vi "探头窗口-6.vi"() -> ()   [LabVIEW 2017]
panel:
  in  "更新数据":T1
  in  "停止信号":bool=TRUE
  out "更新数据？":bool=TRUE
  out "引用-切回列表模式？":refnum<vi>
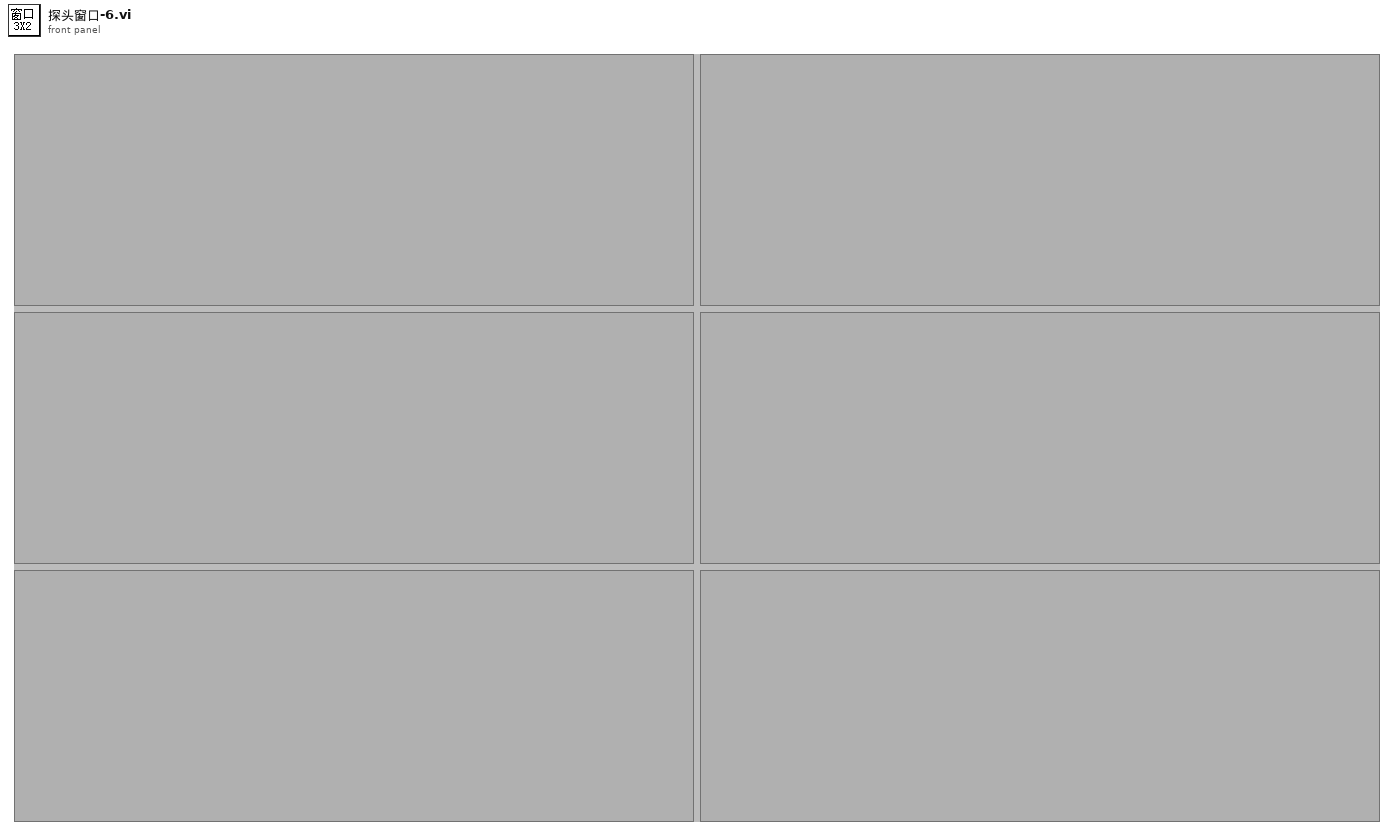
[diagram p1: front panel]
types:
  T1 = cluster{"探头启用状态？":bool[], "测量值":cluster{"X":timestamp, "Y":dbl}[], "限值":cluster{"限值1":dbl, "限值2":dbl, "探头限值":enum16{"一级限值", "二级限值"}}[], "报警状态":enum16{"正常", "一级报警", "二级报警", "累积报警"}[], "探头信息":string[], "累积剂量":cluster{"设备名称":string, "启用累积？":bool, "起始时间":timestamp, "累积剂量":dbl, "累积报警阈值":dbl}[]}
  T2 = cluster{"启用状态？":bool, "测量值":cluster{"X":timestamp, "Y":dbl}, "限值簇":cluster{"限值1":dbl, "限值2":dbl, "探头限值":enum16{"一级限值", "二级限值"}}, "报警状态":enum16{"正常", "一级报警", "二级报警", "累积报警"}, "探头信息":string, "探头地址":i32, "累积剂量":cluster{"设备名称":string, "启用累积？":bool, "起始时间":timestamp, "累积剂量":dbl, "累积报警阈值":dbl}}
  T3 = cluster{"限值1":dbl, "限值2":dbl, "探头限值":enum16{"一级限值", "二级限值"}}
  T4 = cluster{"限值1":dbl, "限值2":dbl, "探头限值":enum16{"一级限值", "二级限值"}}[]
  T5 = cluster{"设备名称":string, "启用累积？":bool, "起始时间":timestamp, "累积剂量":dbl, "累积报警阈值":dbl}[]
  T6 = cluster{"设备名称":string, "启用累积？":bool, "起始时间":timestamp, "累积剂量":dbl, "累积报警阈值":dbl}
  T7 = typedef "eventvkey.ctl" = enum16{"ASCII", "Enter", "Return", "Shift", "Ctrl", "Alt", "Cmd", "Opt", "Caps", "NumLock", "Clear", "Break", "Up", "Down", "Left", "Right", "Insert", "Delete", "Home", "End", "PageUp", "PageDown", "Escape", "Help", "Pause", "ScrollLock", "F1", "F2", "F3", "F4", "F5", "F6", "F7", "F8", "F9", "F10", "F11", "F12", "F13", "F14", "F15", "F16", "F17", "F18", "F19", "F20", "F21", "F22", "F23", "F24", "Play", "VolumeUp", "VolumeDown", "Mute", "Two Byte Char"}
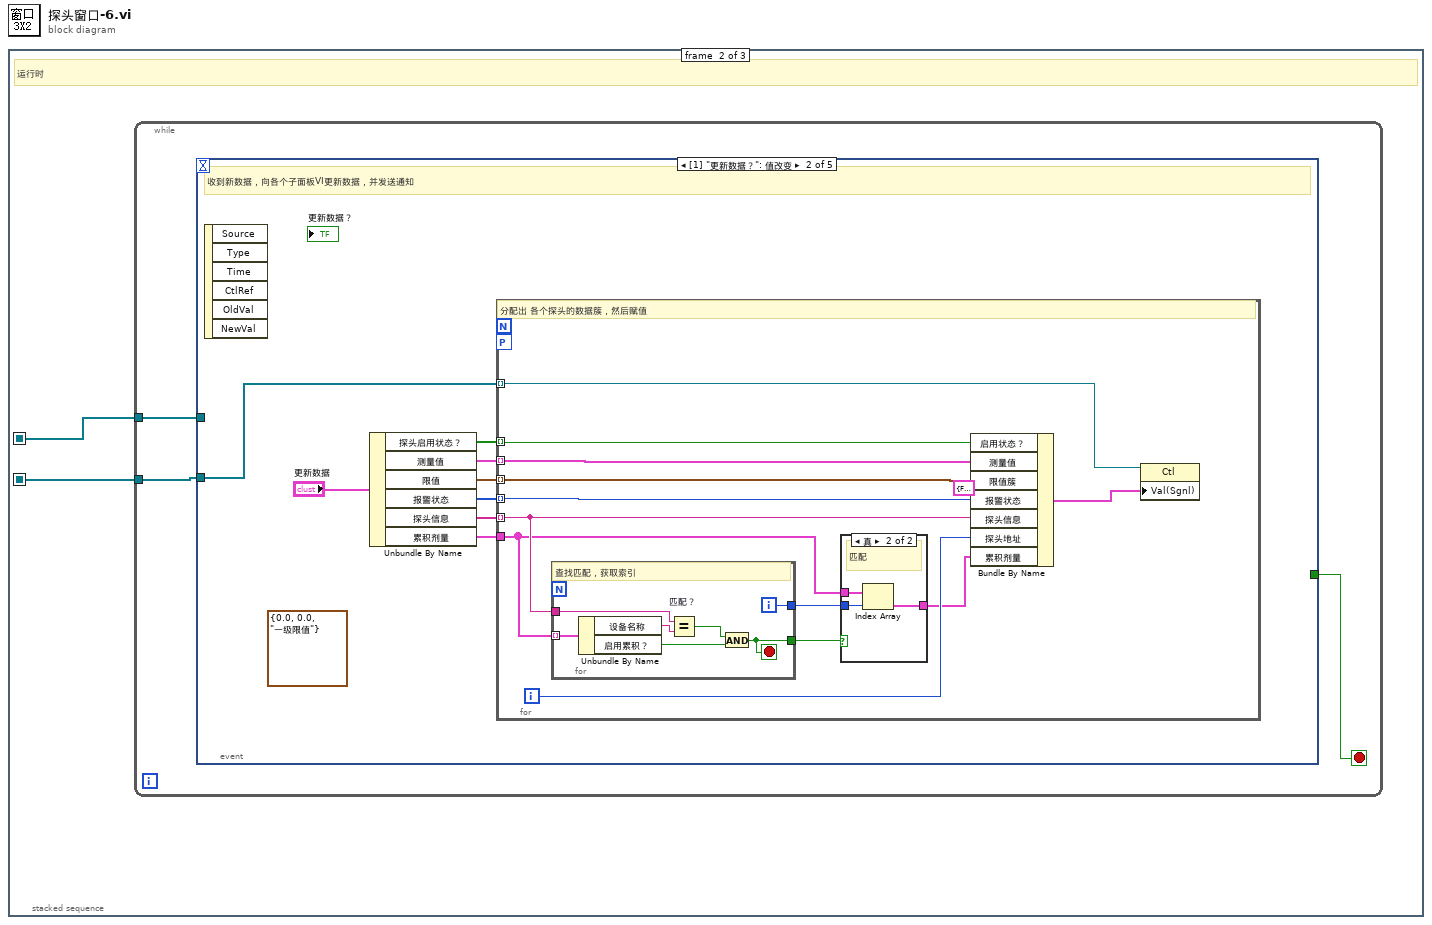
[diagram p0: block diagram]
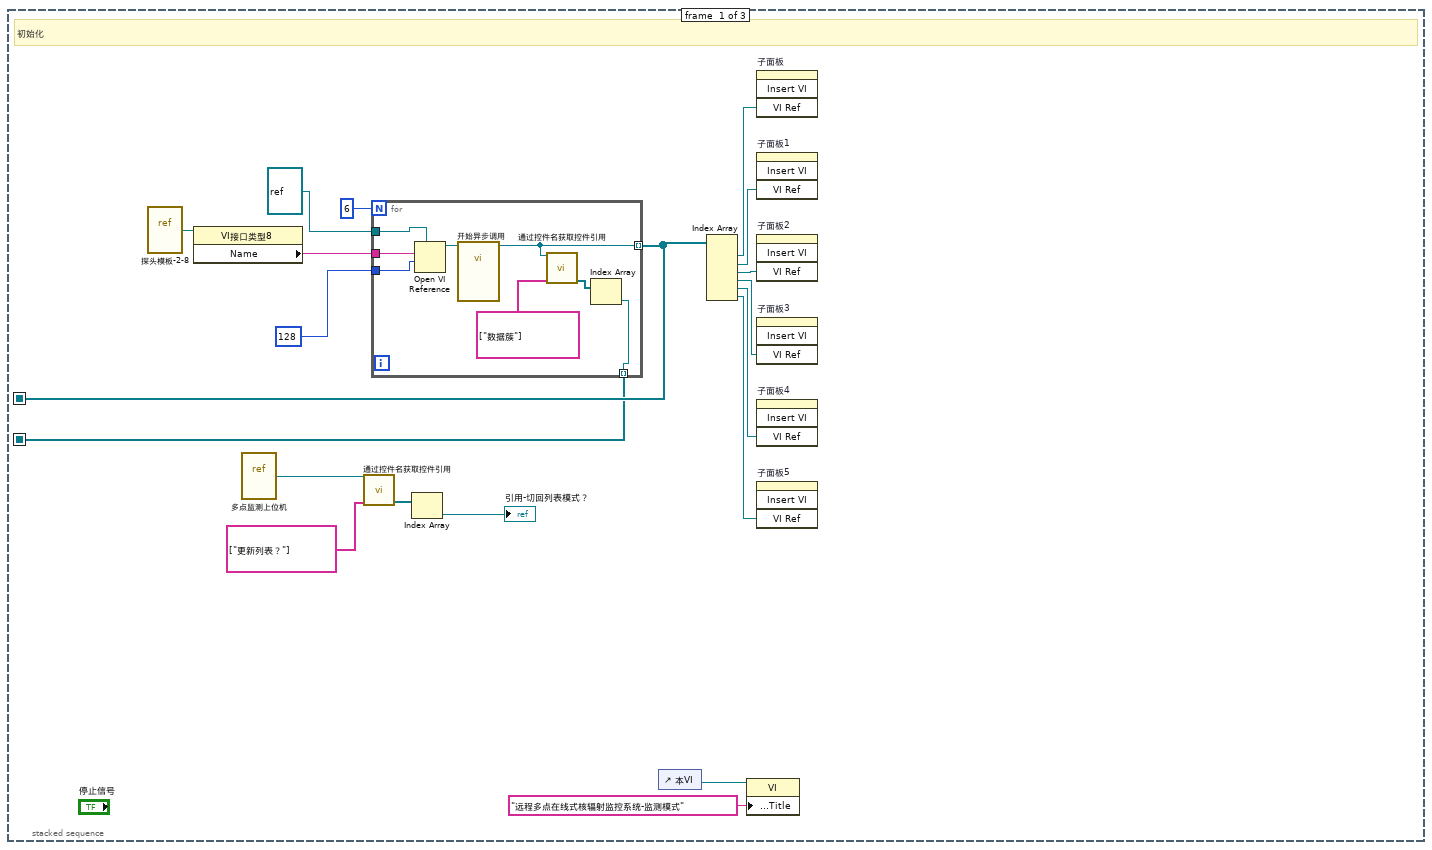
[diagram p2: hidden frame]
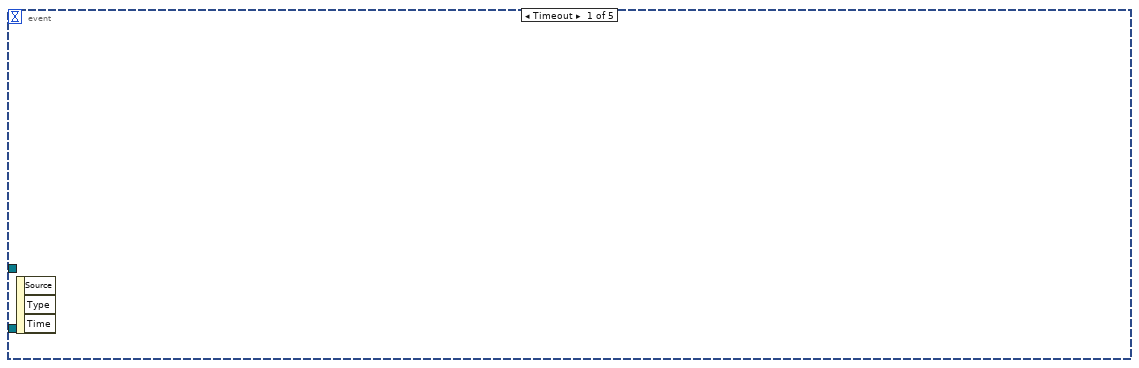
[diagram p3: hidden frame]
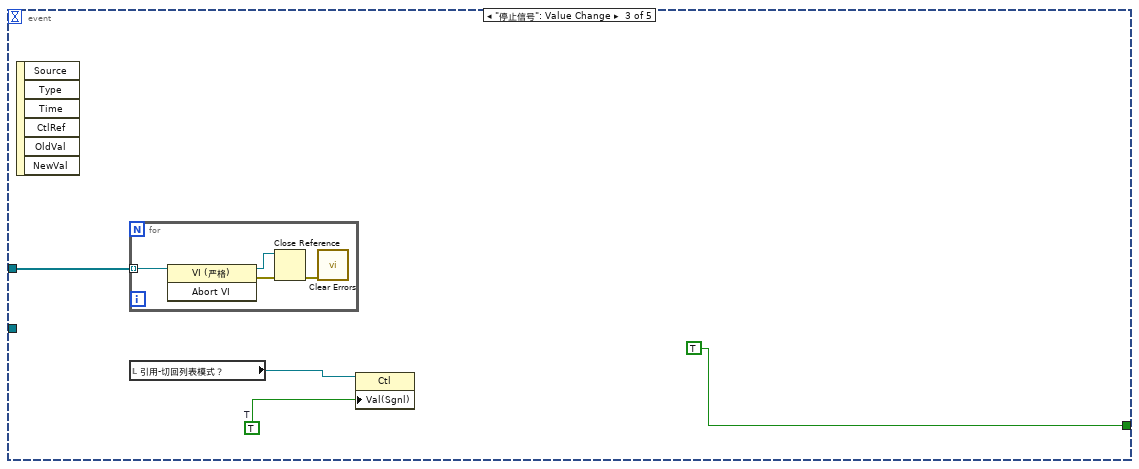
[diagram p5: hidden frame]
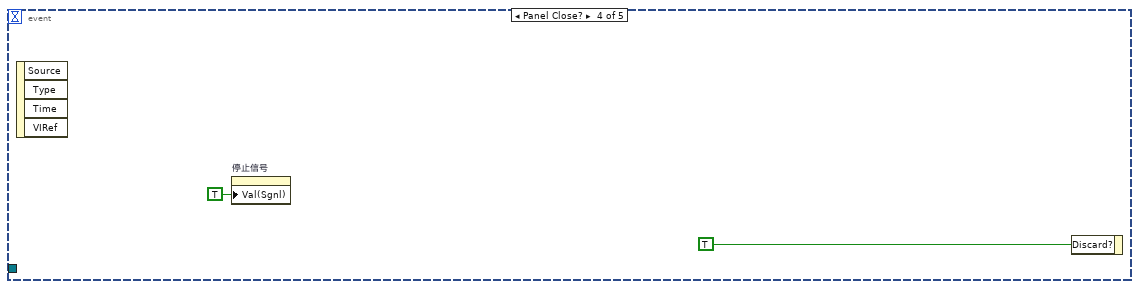
[diagram p6: hidden frame]
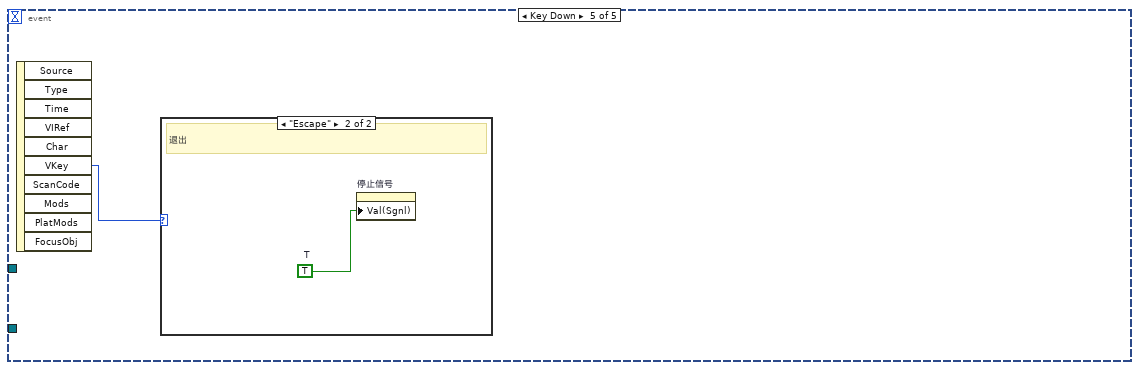
[diagram p7: hidden frame]
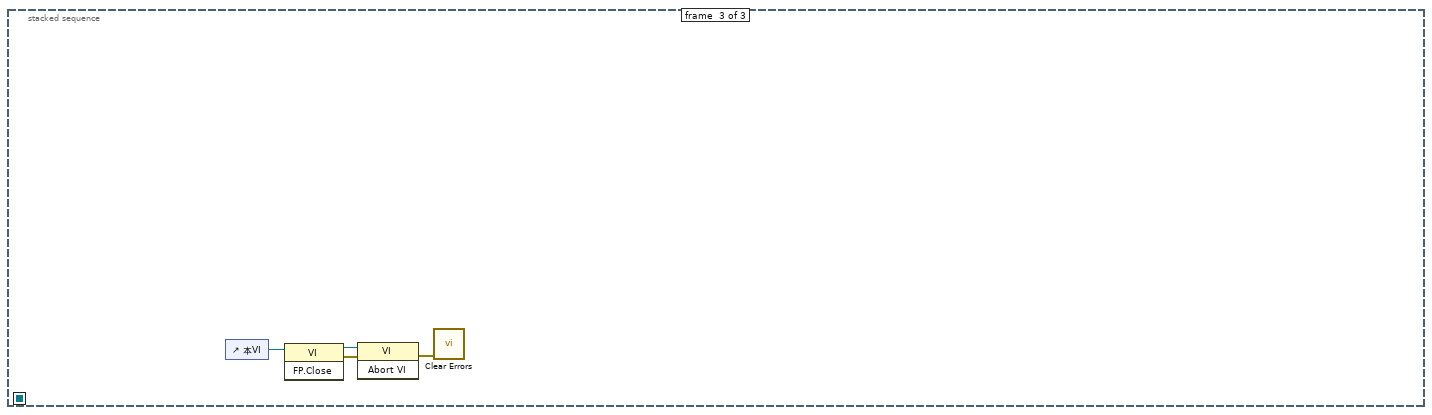
[diagram p9: hidden frame]
diagram:
  n1 = stacked-sequence {
    seq-local: [w15 _ _] -> [_ w29 _]
    seq-local: [w7 _ _] -> [_ w28 _]
    frame #0 {
      # "初始化"
      n2 = vi-ref "探头模板-2-8.vi"() -> (w19:refnum<vi>)
      n3 = property class="VI接口类型8"(reference=w19) -> ("Name"=w18:string)  [unwired: 1 in, 2 out]
      n4 = vi-ref "多点监测上位机.vi"() -> (w3:refnum<vi>)
      n5 = call "通过控件名获取控件引用.vi"("控件名数组"=string[] ["更新列表？"], "VI引用"=w3) -> ("控件引用输出"=w5:refnum<vi>[])  [unwired: 7 in, 2 out]
      n6 = for {
        N: 6 -> [_]
        tunnel: w18 -> [w27]
        tunnel: 128 ("选项") -> [w26]
        tunnel: refnum<vi> refnum ("类型说明符VI引用句柄（仅用于类型）") -> [w25]
        tunnel: [w20] -> w15 mode=indexing
        tunnel: [w21] -> w7 mode=indexing
        n7 = Open VI Reference(type specifier VI Refnum (for type only)=w25, vi path=w27, options=w26) -> (vi reference=w22:refnum<vi>)  [unwired: 3 in, 1 out]
        n8 = call-by-ref "开始异步调用"(reference=w22) -> (reference out=w20:refnum<vi>)  [unwired: 13 in, 1 out]
        n9 = call "通过控件名获取控件引用.vi"("控件名数组"=string[] ["数据簇"], "VI引用"=w20) -> ("控件引用输出"=w24:refnum<vi>[])  [unwired: 7 in, 2 out]
        n10 = Index Array(array=w24) -> (element=w21:refnum<vi>)  [unwired: 1 in]
      }
      n11 = Index Array(array=w5) -> (element=→"引用-切回列表模式？":refnum<vi>)  [unwired: 1 in]
      n12 = control-ref of="本VI"() -> (w2:refnum<vi>)
      n13 = Index Array(array=w15) -> (element #1=w13:refnum<vi>, element #2=w12:refnum<vi>, element #3=w11:refnum<vi>, element #4=w10:refnum<vi>, element #5=w8:refnum<vi>, element #6=w9:refnum<vi>)  [unwired: 6 in]
      n14 = property class="VI"(reference=w2, "Front Panel.Title"="远程多点在线式核辐射监控系统-监测模式" ("前面板窗口:标题")) -> ()  [unwired: 1 in, 2 out]
      n15 = invoke on="子面板" class="子面板" method="Insert VI"("VI Ref"=w13) -> ()  [unwired: 3 in, 4 out]
      n16 = invoke on="子面板1" class="SubPnl" method="Insert VI"("VI Ref"=w12) -> ()  [unwired: 3 in, 4 out]
      n17 = invoke on="子面板2" class="SubPnl" method="Insert VI"("VI Ref"=w11) -> ()  [unwired: 3 in, 4 out]
      n18 = invoke on="子面板3" class="SubPnl" method="Insert VI"("VI Ref"=w10) -> ()  [unwired: 3 in, 4 out]
      n19 = invoke on="子面板4" class="SubPnl" method="Insert VI"("VI Ref"=w8) -> ()  [unwired: 3 in, 4 out]
      n20 = invoke on="子面板5" class="SubPnl" method="Insert VI"("VI Ref"=w9) -> ()  [unwired: 3 in, 4 out]
    }
    frame #1 {
      # "运行时"
      n21 = while {
        tunnel: w29 -> [w31]
        tunnel: w28 -> [w30]
        stop <- w32 stop-if-true
        n22 = event shown="[1] \"更新数据？\": 值改变" {
          selector: _ -> [_ _ _ _ _]
          dyn-events: _ -> [_ _ _ _ _]
          timeout: _ -> [_ _ _ _ _]
          tunnel: [_ _ TRUE ("放弃？") _ _] -> w32
          tunnel: w31 -> [_ _ w66 _ _]
          tunnel: w30 -> [_ w33 _ _ _]
          event Timeout {
            n23 = event-data() -> ()  [unwired: 1 in, 3 out]
          }
          event "更新数据？": Value Change {
            (unwired) T3 {"限值1"=0.0, "限值2"=0.0, "探头限值"=enum."一级限值"} ("探头限值簇")
            # "收到新数据，向各个子面板VI更新数据，并发送通知"
            n24 = event-data() -> ()  [unwired: 1 in, 6 out]
            n25 = Unbundle By Name("更新数据") -> ("探头启用状态？"=w34:bool[], "测量值"=w35:cluster{"X":timestamp, "Y":dbl}[], "限值"=w36:T4, "报警状态"=w37:enum16{"正常", "一级报警", "二级报警", "累积报警"}[], "探头信息"=w38:string[], "累积剂量"=w39:T5)
            n26 = for {
              tunnel: w34 -> [w53] mode=indexing
              tunnel: w35 -> [w52] mode=indexing
              tunnel: w36 -> [w51] mode=indexing
              tunnel: w37 -> [w50] mode=indexing
              tunnel: w38 -> [w45] mode=indexing
              workers-P: _ -> [_]
              tunnel: w33 -> [w48] mode=indexing
              tunnel: w39 -> [w44]
              i -> [w46]
              # "分配出 各个探头的数据簇，然后赋值"
              n27 = for {
                tunnel: w44 -> [w63] mode=indexing
                tunnel: w45 -> [w61]
                tunnel: [w58] -> w43
                tunnel: [w57] -> w42
                i -> [w58]
                stop <- w57 stop-if-true
                # "查找匹配，获取索引"
                n28 = Unbundle By Name(w63) -> ("设备名称"=w62:string, "启用累积？"=w59:bool)
                n29 = Equal? "匹配？"(x=w61, y=w62) -> (x = y?=w60:bool)
                n30 = And(x=w60, y=w59) -> (x .and. y?=w57:bool)
              }
              n31 = case shown="真" w42 {
                tunnel: w44 -> [_ w56]
                tunnel: w43 -> [_ w55]
                tunnel: [_ w54] -> w41
                frame False {
                  # "不匹配"
                }
                frame True {
                  # "匹配"
                  n32 = Index Array(array=w56, index=w55) -> (element=w54:T6)
                }
              }
              n33 = Bundle By Name(cluster=T2 {"启用状态？"=FALSE, "测量值"={"X"=timestamp(0 s since 1904-01-01), "Y"=0.0}, "限值簇"={"限值1"=0.0, "限值2"=0.0, "探头限值"=enum."一级限值"}, "报警状态"=enum."正常", "探头信息"="", "探头地址"=0, "累积剂量"={"设备名称"="", "启用累积？"=FALSE, "起始时间"=timestamp(0 s since 1904-01-01), "累积剂量"=0.0, "累积报警阈值"=0.0}} ("输出簇"), "启用状态？"=w53, "测量值"=w52, "限值簇"=w51, "报警状态"=w50, "探头信息"=w45, "探头地址"=w46, "累积剂量"=w41) -> (w47:T2)
              n34 = property class="Ctl"(reference=w48, "Val(Sgnl)"=w47) -> ()  [unwired: 1 in, 2 out]
            }
          }
          event "停止信号": Value Change {
            w65 = TRUE  # T
            n35 = event-data() -> ()  [unwired: 1 in, 6 out]
            n36 = for {
              tunnel: w66 -> [w71] mode=indexing
              n37 = invoke class="VI (严格)" method="Abort VI"(reference=w71) -> (reference out=w69:refnum<vi>, error out=w70:errorcluster)  [unwired: 2 in, 1 out]
              n38 = Close Reference(reference=w69, error in (no error)=w70) -> (error out=w68:errorcluster)
              n39 = call <vilib>:"Clear Errors.vi"("error in (no error)"=w68) -> ()  [unwired: 5 in, 2 out]
            }
            n40 = local read "引用-切回列表模式？"() -> (w64:refnum<vi>)
            n41 = property class="Ctl"(reference=w64, "Val(Sgnl)"=w65) -> ()  [unwired: 1 in, 2 out]
          }
          event Panel Close? {
            n42 = event-data() -> ()  [unwired: 1 in, 4 out]
            n43 = property on="停止信号" class="Bool (严格)"("Val(Sgnl)"=TRUE ("值(信号)")) -> ()  [unwired: 2 in, 2 out]
            n44 = event-data("Discard?"=TRUE ("放弃？")) -> ()  [unwired: 1 in, 1 out]
          }
          event Key Down {
            n45 = event-data() -> ("VKey"=w74:T7)  [unwired: 1 in, 9 out]
            n46 = case shown="\"Escape\"" w74 {
              frame "ASCII", Default {
              }
              frame "Escape" {
                w75 = TRUE  # T
                # "退出"
                n47 = property on="停止信号" class="Bool (严格)"("Val(Sgnl)"=w75) -> ()  [unwired: 2 in, 2 out]
              }
            }
          }
        }
      }
    }
    frame #2 {
      n48 = control-ref of="本VI"() -> (w79:refnum<vi>)
      n49 = invoke class="VI" method="FP.Close"(reference=w79) -> (reference out=w78:refnum<vi>, error out=w77:errorcluster)  [unwired: 2 in, 1 out]
      n50 = invoke class="VI" method="Abort VI"(reference=w78, error in=w77) -> (error out=w76:errorcluster)  [unwired: 1 in, 2 out]
      n51 = call <vilib>:"Clear Errors.vi"("error in (no error)"=w76) -> ()  [unwired: 5 in, 2 out]
    }
  }
